vi "Str_1D.vi"(4 "Array":string[](array[string])) -> (1 "Const_Str_1D.lvclass":refnum<class "Const_Str_1D.lvclass">)   [LabVIEW 2021, in "Const_Str_1D.lvclass"]
uses:
  Const_Str_1D.lvclass
  Const_Str_1D.lvclass/Const_Str_1D.ctl
  Properties/Write Value.vi
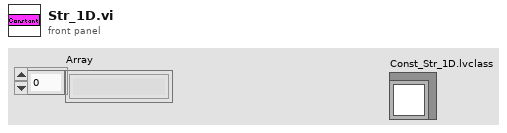
[diagram p1: front panel]
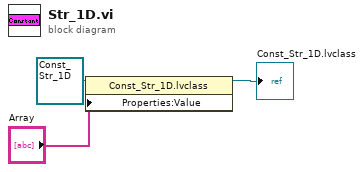
[diagram p0: block diagram]
diagram:
  n1 = property class="Const_Str_1D.lvclass"(reference=refnum<class "Const_Str_1D.lvclass"> refnum ("Const_Str.lvclass"), "Properties:Value"="Array") -> (reference out=→"Const_Str_1D.lvclass":refnum<class "Const_Str_1D.lvclass">)  [unwired: 1 in, 1 out]
